vi "FP Post Build.vi"() -> ()   [LabVIEW 2013]
uses:
  PostBuildSupport (saved for 2013)/PostBuildSupport (2013).lvclass
panel:
  in  "Package Version":string="4.50.1"
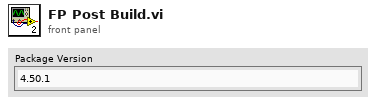
[diagram p1: front panel]
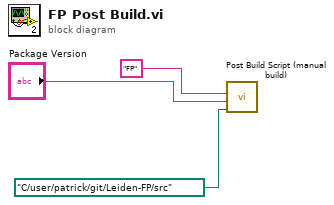
[diagram p0: block diagram]
diagram:
  n1 = call "Post Build Script (manual build).vi"("Package Source Folder"=path "C:/user/patrick/git/Leiden-FP/src", "Package Version"="Package Version", "Product Name"="FP") -> ()  [unwired: 8 in, 1 out]
